vi "Save2Matlab.vi"(0 "Xr":dbl[](array[numeric]), 5 "Yr":dbl[](array[numeric]), 6 "Line":string, 8 "Band touch loose":u32, 9 "Xy":dbl[](array[numeric]), 10 "Band touch win":u32, 11 "Yy":dbl[](array[numeric]), 12 "Path":path, 13 "Xw":dbl[](array[numeric]), 14 "Yw":dbl[](array[numeric]), 15 "error in (no error)":errorcluster) -> (2 "Completed Matlab script":string, 4 "error out":errorcluster)   [LabVIEW 2022 SP3]
doc: "This VI creates a .m file with a specific script\n\nIt has 4 main missions : \n- Adding the X Y coordinates arrays at the top of the code\n- Changing the color of the plots for winning and loosing cases\n- Changing the line style of the plots\n- Adding the sequence's name to the plot's title\n\nNote :\nU32 values of input colors are converted in hexadecimal to be used in Matlab. We need values containing 6 digits.\n\n--/!\\-- WARNING --/!\\-- \n\nThis VI uses a matlab script with temporal variables. It can't be directly used in Matlab because the VI \"Save2Matlab\" has to replaces those variables with some datas.\n\n--/!\\-- WARNING --/!\\-- \n\nInputs :\n- The X and Y arrays for each ball (DBL)\n- The path to the sequence's folder\n- Band touch win (U32)\n- Band touch loose (U32)\n- Line (string)\n- Error in\n\nOutputs :\n- The completed Matlab script (string)\n- Error out"
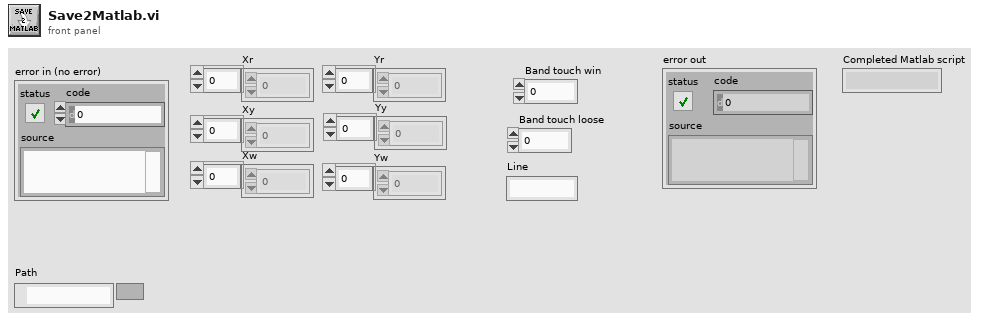
[diagram p1: front panel]
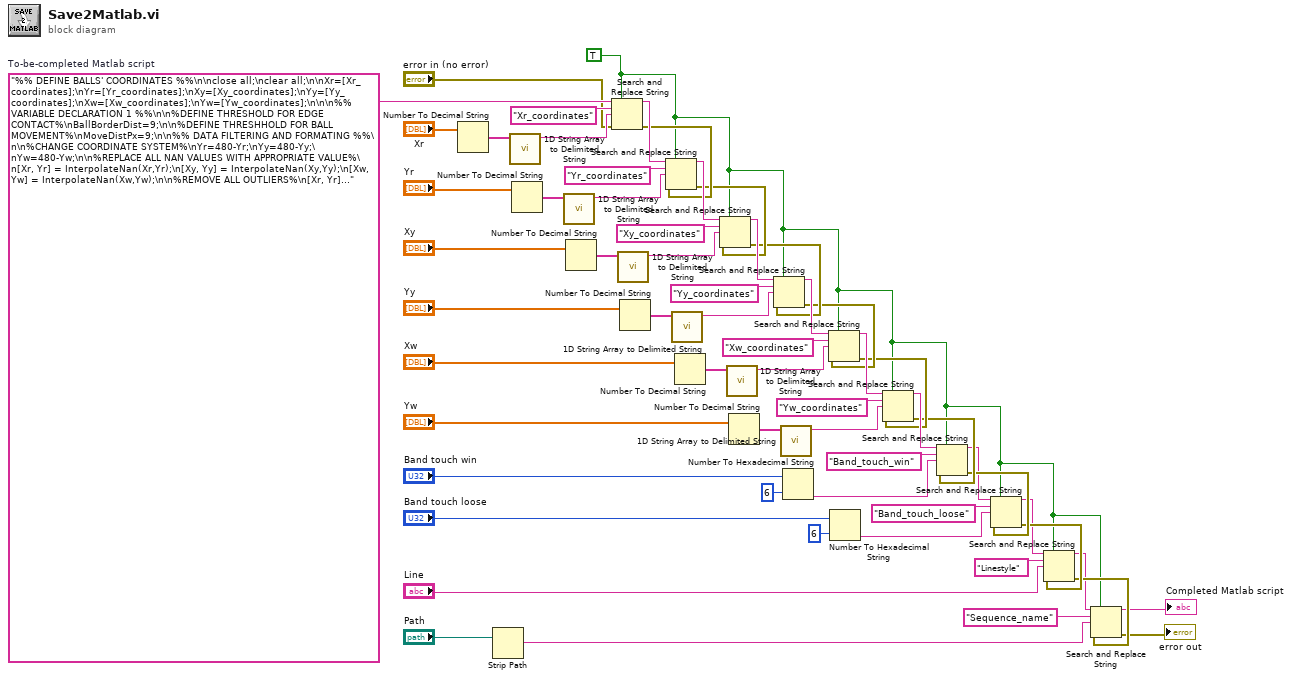
[diagram p0: block diagram]
diagram:
  w1 = TRUE
  w42 = "%% DEFINE BALLS' COORDINATES %%\n\nclose all;\nclear all;\n\nXr=[Xr_coordinates];\nYr=[Yr_coordinates];\nXy=[Xy_coordinates];\nYy=[Yy_coordinates];\nXw=[Xw_coordinates];\nYw=[Yw_coordinates];\n\n\n%% VARIABLE DECLARATION 1 %%\n\n%DEFINE THRESHOLD FOR EDGE CONTACT%\nBallBorderDist=9;\n\n%DEFINE THRESHHOLD FOR BALL MOVEMENT%\nMoveDistPx=9;\n\n%% DATA FILTERING AND FORMATING %%\n\n%CHANGE COORDINATE SYSTEM%\nYr=480-Yr;\nYy=480-Yy;\nYw=480-Yw;\n\n%REPLACE ALL NAN VALUES WITH APPROPRIATE VALUE%\n[Xr, Yr] = InterpolateNan(Xr,Yr);\n[Xy, Yy] = InterpolateNan(Xy,Yy);\n[Xw, Yw] = InterpolateNan(Xw,Yw);\n\n%REMOVE ALL OUTLIERS%\n[Xr, Yr] = RemoveOutlier(Xr,Yr);\n[Xy, Yy] = RemoveOutlier(Xy,Yy);\n[Xw, Yw] = RemoveOutlier(Xw,Yw);\n\n%% COMPUTATION %%\n\n%FIND THE BOUNDARY BOX%\n[Xmin, Xmax, Ymin, Ymax] = GetFrame(Xr,Yr,Xy,Yy,Xw,Yw);\n\n%COMPUTE PATH LENGTH%\nPathLength_r = GetBallPathLength(Xr,Yr);\nPathLength_y = GetBallPathLength(Xy,Yy);\nPathLength_w = GetBallPathLength(Xw,Yw);\n\n%FIND INSTANCES WHEN BALLS TOUCH EDGE%\n[IdxTouch_r]=GetTouchIdx(Xr,Yr,Xmin, Xmax, Ymin, Ymax, BallBorderDist);\n[IdxTouch_y]=GetTouchIdx(Xy,Yy,Xmin, Xmax, Ymin, Ymax, BallBorderDist);\n[IdxTouch_w]=GetTouchIdx(Xw,Yw,Xmin, Xmax, Ymin, Ymax, BallBorderDist);\n\n%FIND BALL MOVE ORDER%\n[FirstBall,SecondBall,LastBall, NbBallsMoved] = GetBallMoveOrder(Xr, Yr, Xy, Yy, Xw, Yw, MoveDistPx);\n\nFirstMoveIdxRed = GetFirstMoveIdx(Xr,Yr, MoveDistPx);\nFirstMoveIdxYellow = GetFirstMoveIdx(Xy,Yy, MoveDistPx);\nFirstMoveIdxWhite = GetFirstMoveIdx(Xw,Yw, MoveDistPx);\n\nSortedvalues = sort([FirstMoveIdxRed FirstMoveIdxYellow FirstMoveIdxWhite]);\nSecondballmoving = Sortedvalues(2);\nif length(Sortedvalues)==2\nelse\nThirdballmoving = Sortedvalues(3);\nend\n\n%% VARIABLE DECLARATION 2 %%\n\n%DEFINE LENGTH AND WIDTH OF BOUNDARY BOX%\nlength_rectangle = Xmax-Xmin;\nwidth_rectangle = Ymax-Ymin;\n\n%DEFIN DATE FOR PLOT%\nnow_time = datetime('now');\ndate = datestr(now_time);\n\n%DEFINE NAME OF SEQUENCE%\nsequence='Sequence_name';\n\n\n%% VICTORY DETECTION %%\n\n%PLAYER DETECTION%\n\nif FirstBall == 1\n    band_touches = IdxTouch_r;\n    if length(Sortedvalues)==2\n    band_touches = band_touches(find(band_touches>=Secondballmoving));\n    else\n    band_touches = band_touches(find(band_touches>=Secondballmoving));\n    band_touches = band_touches(find(band_touches<=Thirdballmoving));\n    FirstBall_color = 'red';\n    end\n\nelseif FirstBall == 2\n    band_touches = IdxTouch_y;\n\n    if length(Sortedvalues)==2\n    band_touches = band_touches(find(band_touches>=Secondballmoving));\n    else\n    band_touches = band_touches(find(band_touches>=Secondballmoving));\n    band_touches = band_touches(find(band_touches<=Thirdballmoving));\n    end\n    FirstBall_color = 'yellow';\n\nelse\n    band_touches = IdxTouch_w;\n    if length(Sortedvalues)==2\n    band_touches = band_touches(find(band_touches>=Secondballmoving));\n    else\n    band_touches = band_touches(find(band_touches>=Secondballmoving));\n    band_touches = band_touches(find(band_touches<=Thirdballmoving));\n    end\n    FirstBall_color = 'white';\n\nend\n%VICTORY CONDITION : WIN%\n\nif length(band_touches)>=3  && NbBallsMoved == 3\n    result = '---WIN---';\n\n%PLOTTING WIN %\nScores_sheet = rectangle('Position',[Xmin Ymin length_rectangle width_rectangle],'EdgeColor','b');\n\n%HOLD ON TO PLOT ON SCORE SHEET%\nhold on\n\n%PLOT ALL THREE BALLS%\nplot(Xr,Yr,'rLinestyle');\nplot(Xy,Yy,'yLinestyle');\nplot(Xw,Yw,'bLinestyle');\n\n%CHANGE PLOT DESCRIPTION%\nset(gca,'XColor', 'none','YColor','none');\naxis([Xmin-20, Xmax+20, Ymin-130, Ymax+20]);%change white zone around the plot\ntitle(['Scores sheet - ' sequence ' - ' date]);\ntext(128, 70, ['Sheet score for the ' FirstBall_color ' ball :'], 'HorizontalAlignment', 'left','FontSize',8);\ntext(128, 50, result, 'HorizontalAlignment', 'left','FontSize',8);\ntext(600, 70, [ num2str(NbBallsMoved) ' ball(s) moved'],'HorizontalAlignment', 'left','FontSize',8);\ntext(600, 50, [ num2str(length(band_touches)) ' band(s) touched'],'HorizontalAlignment', 'left','FontSize',8);\ntext(128, 20, [ 'Red ball distance : ' num2str(PathLength_r) ' px'],'HorizontalAlignment', 'left','FontSize',8);\ntext(128, 0, [ 'Yellow ball distance : ' num2str(PathLength_y) ' px'],'HorizontalAlignment', 'left','FontSize',8);\ntext(128, -20, [ 'White ball distance : ' num2str(PathLength_w) ' px'],'HorizontalAlignment', 'left','FontSize',8);\n\n%MARK THE BALLS' INITIAL POSTION%\nFr = plot(Xr(1), Yr(1), \"hexagram\",'Color','r');\nFr.MarkerSize = 15;\nFy = plot(Xy(1), Yy(1), \"hexagram\",'Color','y');\nFy.MarkerSize = 15;\nFw = plot(Xw(1), Yw(1), \"hexagram\",'Color','b');\nFw.MarkerSize = 15;\n\n%MARK BAND CONTACTS%\nif FirstBall == 1\nrb = plot(Xr(band_touches), Yr(band_touches), \"o\", 'Color','#Band_touch_win');\nrb.MarkerSize = 15;\nelseif FirstBall == 2\nrb = plot(Xy(band_touches), Yy(band_touches), \"o\", 'Color','#Band_touch_win');\nrb.MarkerSize = 15;\nelse FirstBall == 3\nrb = plot(Xw(band_touches), Yw(band_touches), \"o\", 'Color','#Band_touch_win');\nrb.MarkerSize = 15;\nend\nsaveas(gcf,'ScoresheetSequence_name.pdf')\n%END PLOT%\nhold off;\n\n\n%VICTORY CONDITION : LOOSE%\nelse\n    result = '---LOOSE---';\n\n%PLOTTING LOOSE %\nScores_sheet = rectangle('Position',[Xmin Ymin length_rectangle width_rectangle],'EdgeColor','b');\n\n%HOLD ON TO PLOT ON SCORE SHEET%\nhold on\n\n%PLOT ALL THREE BALLS%\nplot(Xr,Yr,'rLinestyle');\nplot(Xy,Yy,'yLinestyle');\nplot(Xw,Yw,'bLinestyle');\n\n%CHANGE PLOT DESCRIPTION%\nset(gca,'XColor', 'none','YColor','none');\naxis([Xmin-20, Xmax+20, Ymin-130, Ymax+20]);%change white zone around the plot\ntitle(['Scores sheet - ' sequence ' - ' date]);\ntext(128, 70, ['Sheet score for the ' FirstBall_color ' ball :'], 'HorizontalAlignment', 'left','FontSize',8);\ntext(128, 50, result, 'HorizontalAlignment', 'left','FontSize',8);\ntext(600, 70, [ num2str(NbBallsMoved) ' ball(s) moved'],'HorizontalAlignment', 'left','FontSize',8);\ntext(600, 50, [ num2str(length(band_touches)) ' band(s) touched'],'HorizontalAlignment', 'left','FontSize',8);\ntext(128, 20, [ 'Red ball distance : ' num2str(PathLength_r) ' px'],'HorizontalAlignment', 'left','FontSize',8);\ntext(128, 0, [ 'Yellow ball distance : ' num2str(PathLength_y) ' px'],'HorizontalAlignment', 'left','FontSize',8);\ntext(128, -20, [ 'White ball distance : ' num2str(PathLength_w) ' px'],'HorizontalAlignment', 'left','FontSize',8);\n\n%MARK THE BALLS' INITIAL POSTION%\nFr = plot(Xr(1), Yr(1), \"hexagram\",'Color','r');\nFr.MarkerSize = 15;\nFy = plot(Xy(1), Yy(1), \"hexagram\",'Color','y');\nFy.MarkerSize = 15;\nFw = plot(Xw(1), Yw(1), \"hexagram\",'Color','b');\nFw.MarkerSize = 15;\n\n%MARK BAND CONTACTS%\nif FirstBall == 1\nif isempty(Xr(band_touches))\nelse\nrb = plot(Xr(band_touches), Yr(band_touches), \"o\", 'Color','#Band_touch_loose');\nrb.MarkerSize = 15;\nend\nelseif FirstBall == 2\nif isempty(Xy(band_touches))\nelse\nrb = plot(Xy(band_touches), Yy(band_touches), \"o\", 'Color','#Band_touch_loose');\nrb.MarkerSize = 15;\nend\nelse FirstBall == 3\nif isempty(Xw(band_touches))\nelse\nrb = plot(Xw(band_touches), Yw(band_touches), \"o\", 'Color','#Band_touch_loose');\nrb.MarkerSize = 15;\nend\nend\nsaveas(gcf,'ScoresheetSequence_name.pdf')\nhold off;\nend\n\n%% DECLARING FUNCTIONS %%\n\nfunction [FirstBall,SecondBall,LastBall, NbBallsMoved] = GetBallMoveOrder(Xr, Yr, Xy, Yy, Xw, Yw, MoveDistPx)\n%TLDR: FIND IN WHICH ORDER THE BALLS MOVED%\n\n% INPUTS:  - ALL OF THE BALLS' COORDINATES(Xr, Yr, Xy, Yy, Xw, Yw)\n%          - THRESHOLD TO DETECT BALL MOVEMENT(MoveDistPx)%\n\n% OUTPUTS: - ID OF THE FIRST BALL THAT MOVED (FirstBall)\n%          - ID OF THE FIRST BALL THAT MOVED (SecondBall)\n%          - ID OF THE FIRST BALL THAT MOVED (LastBall)\n%          - A COUNT OF HOW MANY BALLS MOVED (NbBallsMoved)%\n  \n%FETCHING FIRST MOVE ID AND DISTANCE MOVED FROM GetForstMoveIdx%\n[IdR, DistR] = GetFirstMoveIdx(Xr,Yr, MoveDistPx);\n[IdY, DistY] = GetFirstMoveIdx(Xy,Yy, MoveDistPx);\n[IdW, DistW] = GetFirstMoveIdx(Xw,Yw, MoveDistPx);\n\n%COUNTS THE NUMBER OF BALLS THAT MOVED%\nId = [IdR IdY IdW];\nNbBallsMoved = length(Id);\n\nif NbBallsMoved == 3\n%CREATE A TEMPORARY MATRIX TO STORE THE FIRST MOVE ID, FIRST MOVE DISTANCE AND BALL ID OF EACH BALL%\nTempMatrix = [IdR -DistR 1; IdY -DistY 2; IdW -DistW 3];\n\n%SORTS TO FIND FIRST MOVE ID ORDER (USES FIRST MOVE DISTANCE IN CASE OF DRAW)%\nTempMatrix = sortrows(TempMatrix);\n\n%DEFINE OUTPUT VALUES%\nFirstBall = TempMatrix(1,3);\nSecondBall = TempMatrix(2,3);\nLastBall = TempMatrix(3,3);\n\nelseif NbBallsMoved == 2\n\n\nif DistR == 0\n\n%CREATE A TEMPORARY MATRIX TO STORE THE FIRST MOVE ID, FIRST MOVE DISTANCE AND BALL ID OF EACH BALL%\nTempMatrix = [IdY -DistY 2; IdW -DistW 3];\n\n%SORTS TO FIND FIRST MOVE ID ORDER (USES FIRST MOVE DISTANCE IN CASE OF DRAW)%\nTempMatrix = sortrows(TempMatrix);\n\nFirstBall = TempMatrix(1,3);\nSecondBall = TempMatrix(2,3);\nLastBall = 1;\n\nelseif DistW == 0\n\n%CREATE A TEMPORARY MATRIX TO STORE THE FIRST MOVE ID, FIRST MOVE DISTANCE AND BALL ID OF EACH BALL%\nTempMatrix = [IdR -DistR 1; IdY -DistY 2];\n\n%SORTS TO FIND FIRST MOVE ID ORDER (USES FIRST MOVE DISTANCE IN CASE OF DRAW)%\nTempMatrix = sortrows(TempMatrix);\n\nFirstBall = TempMatrix(1,3);\nSecondBall = TempMatrix(2,3);\nLastBall = 3;\n\nelse\n\n%CREATE A TEMPORARY MATRIX TO STORE THE FIRST MOVE ID, FIRST MOVE DISTANCE AND BALL ID OF EACH BALL%\nTempMatrix = [IdR -DistR 1; IdW -DistW 3];\n\n%SORTS TO FIND FIRST MOVE ID ORDER (USES FIRST MOVE DISTANCE IN CASE OF DRAW)%\nTempMatrix = sortrows(TempMatrix);\n\nFirstBall = TempMatrix(1,3);\nSecondBall = TempMatrix(2,3);\nLastBall = 2;\nend\n\nend\n\nend\nfunction PathLength=GetBallPathLength(X,Y)\n%TLDR: FIND TOTAL PATH LENGTH%\n\n% INPUTS:  - COORDINATES OF ONE BALL(X,Y)%\n\n% OUTPUTS: - PATHLENGTH (PathLength)%\n\n%COMPUTE THE DIFFENCE IN BETWEEN EACH SUCCESSIVE VALUE OF X AND THEN Y%\nX1=diff(X);\nY1=diff(Y);\n\n%USE PYTHAGOREAN THEOREM TO COMPUTE DISTANCE THE BALL MOVED BETWEEN EACH SUCCESIVE FRAME%\nS=sqrt(X1.^2+Y1.^2);\n\n%SUM ALL THE INDIVIDUAL MOVEMENTS TO FIND THE TOTAL PATHLENGTH%\nPathLength=sum(S);\nif PathLength <= 9\n    PathLength = 0;\nend\nend\n\nfunction [FirstMoveIdx, Dist]=GetFirstMoveIdx(X,Y, MoveDistPx)\n%TLDR: FIND THE THE FRAME AT WHICH A BALL FIRST MOVES%\n\n% INPUTS:  - COORDINATES OF ONE BALL(X,Y)\n%          - THRESHOLD TO DETECT BALL MOVEMENT(MoveDistPx)%\n\n% OUTPUTS: - FRAME AT WHICH THE BALL MOVED (FirstMoveIdx)\n%          - DISTANCE THE BALL MOVED INTIALLY MOVED (Dist)%\n\n%DIFFERENCE IN BETWEEN THE FIRST VALUE OF X AND ALL THE OTHER VALUES OF X%\ndx = X(1)-X;\n\n%DIFFERENCE IN BETWEEN THE FIRST VALUE OF Y AND ALL THE OTHER VALUES OF Y%\ndy = Y(1)-Y;\n\n%COMPUTE THE MOVE DISTANCE IN BETWEEN THE FIRST FRAME AND EVERY OTHER FRAME%\nS = sqrt(dx.^2 + dy.^2);\n\n%CREATE TEMPORARY MATRIX WHICH STORES EVERY FRAME WHERE THE BALL MOVEMENT PASSED THE THRESHHOLD%\nTempMatrix = find(S > MoveDistPx);\n\n%FINDS THE FIRST FRAME WHERE THE BALL MOVED%\nif isempty(TempMatrix)\nDist = 0;  \nFirstMoveIdx = [];\nelse\nFirstMoveIdx = TempMatrix(1);\n%COMPUTE INNITIAL MOVE DISTANCE%\nDist = sqrt((X(FirstMoveIdx)-X(FirstMoveIdx-1))^2+(Y(FirstMoveIdx)-Y(FirstMoveIdx-1))^2)\nend\nend\n\nfunction [Xmin, Xmax, Ymin, Ymax] = GetFrame(Xr,Yr,Xy,Yy,Xw,Yw)\n%TLDR: FIND THE OUTLINE OF THE TABLE%\n\n% INPUTS:  - ALL OF THE BALLS' COORDINATES(Xr, Yr, Xy, Yy, Xw, Yw)%\n\n% OUTPUTS: - ALL OF THE EDGES OF THE TABLE (Xmin, Xmax, Ymin, Ymax)%\n\n%FIND THE SMALLEST VALUES OF X%\nXrmin = min(Xr);\nXymin = min(Xy);\nXwmin = min(Xw);\nXmin = min([Xrmin Xymin Xwmin]);\n\n%FIND THE BIGGEST VALUES OF X%\nXrmax = max(Xr);\nXymax= max(Xy);\nXwmax = max(Xw);\nXmax = max([Xrmax Xymax Xwmax]);\n\n%FIND THE SMALLEST VALUES OF Y%\nYrmin = min(Yr);\nYymin = min(Yy);\nYwmin = min(Yw);\nYmin = min([Yrmin Yymin Ywmin]);\n\n%FIND THE BIGGEST VALUES OF Y%\nYrmax = max(Yr);\nYymax = max(Yy);\nYwmax = max(Yw);\nYmax = max([Yrmax Yymax Ywmax]);\nend\n\nfunction [IdxTouch]=GetTouchIdx(X,Y,Xmin, Xmax, Ymin, Ymax, BallBorderDist)\n%TLDR: FIND FRAMES WHEN BALLS MAKE CONTACT WITH EDGE%\n\n% INPUTS:  - COORDINATES OF ONE BALL(X,Y)\n%          - THRESHOLD TO DETECT CONTACT (BallBorderDist)\n%          - ALL OF THE EDGES OF THE TABLE (Xmin, Xmax, Ymin, Ymax)%\n\n% OUTPUTS: - ALL FRAMES WHEN BALL TOUCHED EDGE (FirstBall)%\n\n%RIGHT EDGE\n%FIND ALL FRAMES WHERE BALL IS BESIDE EDGE%\nDiffXmax = Xmax-X;\ncbt = find(DiffXmax <= BallBorderDist);\n\n%CHECKS IF BALL DID NOT MAKE CONTACT%\nif isempty(cbt)\n    IdxTouchXmax = [];\n\nelse\n    %REMOVES FIRST FRAME FROM IDS WHEN BALL MAKES CONTACT%\n    if cbt(1) == 1\n        cbt(1) = []; \n    end\n\n    %REMOVE SUCCESSIVE FRAMES%\n    Cons = diff(cbt);\n    IdCons = find(Cons == 1);\n    IdCons = IdCons + 1;\n    cbt(:,IdCons) = [];\n\n    %STORE IDS%\n    IdxTouchXmax = cbt;%matrice des index où la boule touche Xmax\nend\n\n%LEFT EDGE\n%FIND ALL FRAMES WHERE BALL IS BESIDE EDGE%\nDiffXmin = X-Xmin;\ncbt = find(DiffXmin <= BallBorderDist);\n\n%CHECKS IF BALL DID NOT MAKE CONTACT%\nif isempty(cbt)\n    IdxTouchXmin = [];\n\nelse\n    %REMOVES FIRST FRAME FROM IDS WHEN BALL MAKES CONTACT%\n    if cbt(1) == 1\n        cbt(1) = []; \n    end\n\n    %REMOVE SUCCESSIVE FRAMES%\n    Cons = diff(cbt);\n    IdCons = find(Cons == 1);\n    IdCons = IdCons + 1;\n    cbt(:,IdCons) = [];\n\n    %STORE IDS%\n    IdxTouchXmin = cbt;%matrice des index où la boule touche Xmax\nend\n\n%TOP EDGE\n%FIND ALL FRAMES WHERE BALL IS BESIDE EDGE%\nDiffYmax = Ymax-Y;\ncbt = find(DiffYmax <= BallBorderDist);\n\n%CHECKS IF BALL DID NOT MAKE CONTACT%\nif isempty(cbt)\n    IdxTouchYmax = [];\n\nelse\n    %REMOVES FIRST FRAME FROM IDS WHEN BALL MAKES CONTACT%\n    if cbt(1) == 1\n        cbt(1) = []; \n    end\n\n    %REMOVE SUCCESSIVE FRAMES%\n    Cons = diff(cbt);\n    IdCons = find(Cons == 1);\n    IdCons = IdCons + 1;\n    cbt(:,IdCons) = [];\n\n    %STORE IDS%\n    IdxTouchYmax = cbt;%matrice des index où la boule touche Xmax\nend\n\n%BOTTOM EDGE\n%FIND ALL FRAMES WHERE BALL IS BESIDE EDGE%\nDiffYmin = Y-Ymin;\ncbt = find(DiffYmin <= BallBorderDist);\n\n%CHECKS IF BALL DID NOT MAKE CONTACT%\nif isempty(cbt)\n    IdxTouchYmin = [];\n\nelse\n    %REMOVES FIRST FRAME FROM IDS WHEN BALL MAKES CONTACT%\n    if cbt(1) == 1\n        cbt(1) = []; \n    end\n\n    %REMOVE SUCCESSIVE FRAMES%\n    Cons = diff(cbt);\n    IdCons = find(Cons == 1);\n    IdCons = IdCons + 1;\n    cbt(:,IdCons) = [];\n\n    %STORE IDS%\n    IdxTouchYmin = cbt;%matrice des index où la boule touche Xmax\nend\n\nIdxTouch = sort([IdxTouchXmin IdxTouchXmax IdxTouchYmin IdxTouchYmax]);\n\nend\n\nfunction [X,Y]=InterpolateNan(X,Y)\n%TLDR: FILL MISSING VALUES WITH NEXT VALUE OR PREVIOUS VALUE IF LAST VALUE%\n\n% INPUTS:  - COORDINATES OF ONE BALL(X,Y)%\n\n% OUTPUTS: - COORDINATES OF ONE BALL(X,Y)%\n\nX=fillmissing(X,'next');\nY=fillmissing(Y,'next');\nX=fillmissing(X,'previous');\nY=fillmissing(Y,'previous');\nend\n\nfunction [X,Y]=RemoveOutlier(X,Y)\n%TLDR: REMOVE OUTLIER BY WAY OF A MOVING MEDIAN%\n\n% INPUTS:  - COORDINATES OF ONE BALL(X,Y)%\n\n% OUTPUTS: - COORDINATES OF ONE BALL(X,Y)%\n\n%FIND OUTLIERS%\nXOutlier = isoutlier(X,\"movmedian\",10);\nIdOutlierX = find(XOutlier);\nYOutlier = isoutlier(Y,\"movmedian\",10);\nIdOutlierY = find(YOutlier);\nIdOutlier = intersect(IdOutlierX, IdOutlierY);\n\n%CHECKS IF THERE IS ANY OUTLIER\nif isempty(IdOutlier)\n\n%REMOVES FIRST FRAME FROM OUTLIERS%\nelse\n\n    if IdOutlier(1) == 1\n    IdOutlier(1) = [];\n    end\n\n%REPLACE OUTLIERS WITH PREVIOUS NON OUTLIER VALUE%\nPrevIdOutlier = IdOutlier - 1;\nX(IdOutlier)= X(PrevIdOutlier);\nY(IdOutlier)= Y(PrevIdOutlier);\nend\nend"  # To-be-completed Matlab script
  n1 = Number To Decimal String(number="Xr") -> (decimal integer string=w60:string[])  [unwired: 1 in]
  n2 = Strip Path(path="Path") -> (name=w7:string)  [unwired: 1 out]
  n3 = call <vilib>:"1D String Array to Delimited String.vi"("string array"=w60) -> ("delimited string"=w59:string)  [unwired: 10 in]
  n4 = Number To Decimal String(number="Yr") -> (decimal integer string=w57:string[])  [unwired: 1 in]
  n5 = call <vilib>:"1D String Array to Delimited String.vi"("string array"=w57) -> ("delimited string"=w56:string)  [unwired: 10 in]
  n6 = Number To Decimal String(number="Xy") -> (decimal integer string=w49:string[])  [unwired: 1 in]
  n7 = Search and Replace String(replace all?=w1, input string=w42, search string="Xr_coordinates", replace string=w59, error in="error in (no error)") -> (result string=w41:string, error out=w29:errorcluster)  [unwired: 3 in, 2 out]
  n8 = call <vilib>:"1D String Array to Delimited String.vi"("string array"=w49) -> ("delimited string"=w50:string)  [unwired: 10 in]
  n9 = Number To Decimal String(number="Yy") -> (decimal integer string=w52:string[])  [unwired: 1 in]
  n10 = Search and Replace String(replace all?=w1, input string=w41, search string="Yr_coordinates", replace string=w56, error in=w29) -> (result string=w40:string, error out=w28:errorcluster)  [unwired: 3 in, 2 out]
  n11 = call <vilib>:"1D String Array to Delimited String.vi"("string array"=w52) -> ("delimited string"=w53:string)  [unwired: 10 in]
  n12 = Number To Decimal String(number="Xw") -> (decimal integer string=w48:string[])  [unwired: 1 in]
  n13 = Search and Replace String(replace all?=w1, input string=w40, search string="Xy_coordinates", replace string=w50, error in=w28) -> (result string=w39:string, error out=w27:errorcluster)  [unwired: 3 in, 2 out]
  n14 = call <vilib>:"1D String Array to Delimited String.vi"("string array"=w48) -> ("delimited string"=w47:string)  [unwired: 10 in]
  n15 = Number To Decimal String(number="Yw") -> (decimal integer string=w45:string[])  [unwired: 1 in]
  n16 = Search and Replace String(replace all?=w1, input string=w39, search string="Yy_coordinates", replace string=w53, error in=w27) -> (result string=w38:string, error out=w26:errorcluster)  [unwired: 3 in, 2 out]
  n17 = call <vilib>:"1D String Array to Delimited String.vi"("string array"=w45) -> ("delimited string"=w44:string)  [unwired: 10 in]
  n18 = Number To Hexadecimal String(1:i16 6 ("width (-)"), 2:"Band touch win") -> (0:w11:string)
  n19 = Search and Replace String(replace all?=w1, input string=w38, search string="Xw_coordinates", replace string=w47, error in=w26) -> (result string=w37:string, error out=w25:errorcluster)  [unwired: 3 in, 2 out]
  n20 = Number To Hexadecimal String(1:i16 6 ("width (-)"), 2:"Band touch loose") -> (0:w12:string)
  n21 = Search and Replace String(replace all?=w1, input string=w37, search string="Yw_coordinates", replace string=w44, error in=w25) -> (result string=w30:string, error out=w24:errorcluster)  [unwired: 3 in, 2 out]
  n22 = Search and Replace String(replace all?=w1, input string=w30, search string="Band_touch_win", replace string=w11, error in=w24) -> (result string=w18:string, error out=w23:errorcluster)  [unwired: 3 in, 2 out]
  n23 = Search and Replace String(replace all?=w1, input string=w18, search string="Band_touch_loose", replace string=w12, error in=w23) -> (result string=w17:string, error out=w20:errorcluster)  [unwired: 3 in, 2 out]
  n24 = Search and Replace String(replace all?=w1, input string=w17, search string="Linestyle", replace string="Line", error in=w20) -> (result string=w6:string, error out=w9:errorcluster)  [unwired: 3 in, 2 out]
  n25 = Search and Replace String(replace all?=w1, input string=w6, search string="Sequence_name", replace string=w7, error in=w9) -> (result string=→"Completed Matlab script":string, error out=→"error out":errorcluster)  [unwired: 3 in, 2 out]
